vi "ErrorCatcher.vi"(8 "error in":errorcluster, 11 "input String":string) -> (0 "error out":errorcluster)   [LabVIEW 2013]
panel:
  out "concatenated string":string
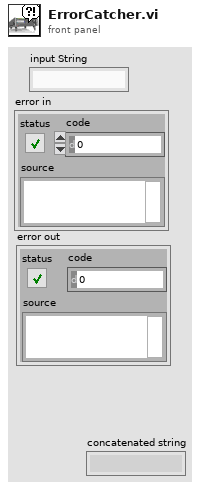
[diagram p1: front panel]
types:
  T1 = cluster{"output string":string, "output string":string}
  T2 = cluster{"output string":string, "output string":string}[]
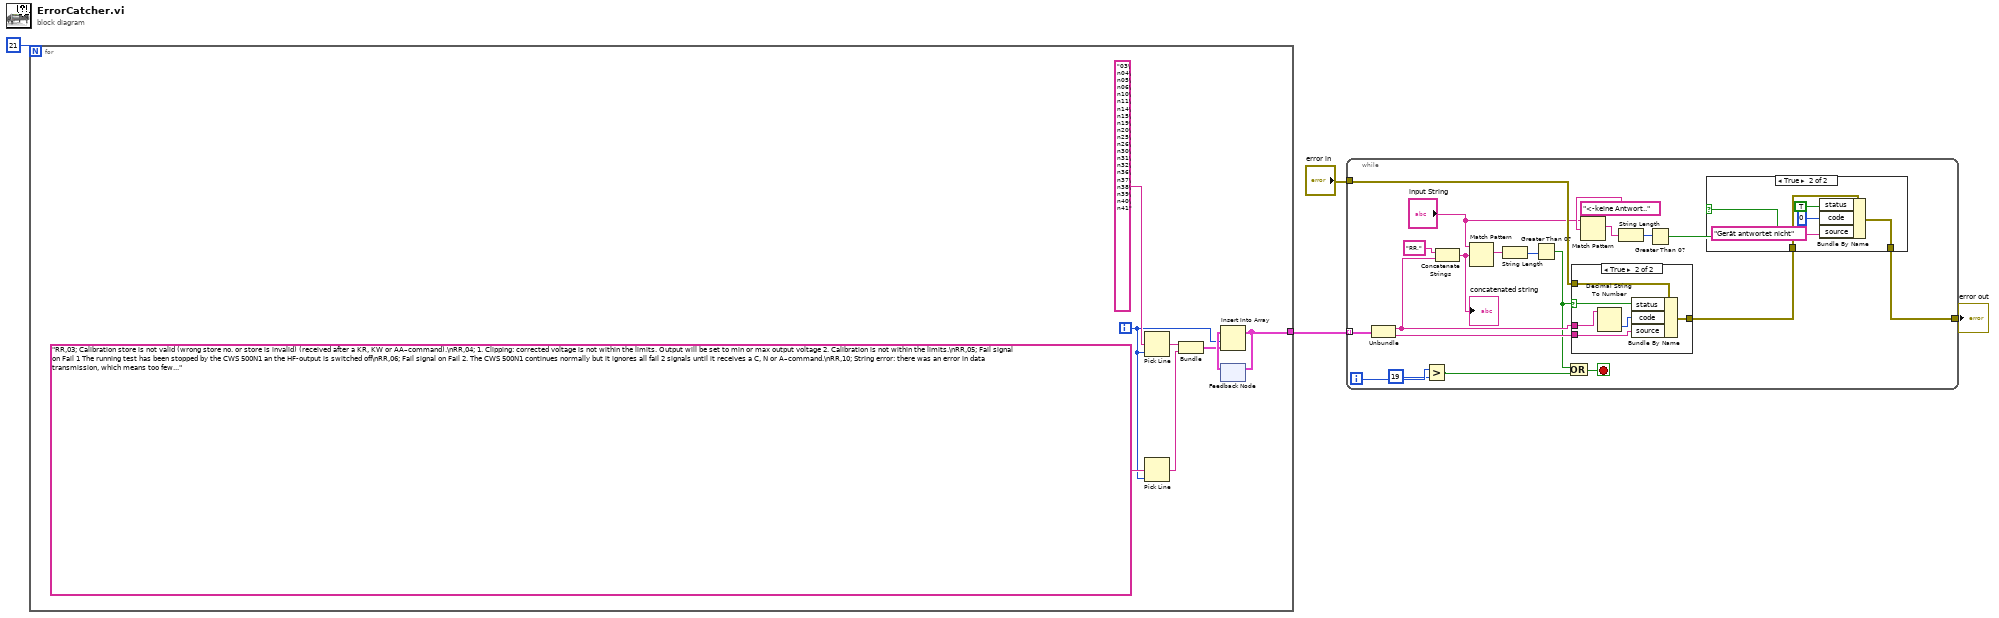
[diagram p0: block diagram]
diagram:
  n1 = for {
    N: 21 -> [_]
    tunnel: [w5] -> w4
    i -> [w7]
    n2 = Pick Line(multi-line string="03\n04\n05\n06\n10\n11\n14\n15\n19\n20\n25\n26\n30\n31\n32\n36\n37\n38\n39\n40\n41", line index=w7) -> (output string=w6:string)  [unwired: 1 in]
    n3 = Pick Line(multi-line string="RR,03; Calibration store is not valid (wrong store no. or store is invalid) (received after a KR, KW or AA–command).\nRR,04; 1. Clipping: corrected voltage is not within the limits. Output will be set to min or max output voltage 2. Calibration is not within the limits.\nRR,05; Fail signal on Fail 1 The running test has been stopped by the CWS 500N1 an the HF-output is switched off\nRR,06; Fail signal on Fail 2. The CWS 500N1 continues normally but it ignores all fail 2 signals until it receives a C, N or A–command.\nRR,10; String error: there was an error in data transmission, which means too few or too many characters or the command is not acceptable.\nRR,11; Test start is not possible or the test has been stopped because TEST ON is not switched on.\nRR,14; One or several values are limited by the CWS 500N1. The parameters are set to their minimum.\nRR,15; Check sum error. The whole command should be sent again.\nRR,19; Internal communication error. Turn off and on the CWS 500N1.\nRR,20; Not correctable limitation error. One or more parameter can not be set to its minimum.\nRR,25; The received calibration data are corrupt (Min-value or Max-value are incorrect or element-no. 265 is not set to 255) (received after a KW–command).\nRR,26; Error on internal Eeprom (write-protected, memory busy) The test routine has been finished correctly using the current monitor. •  This answer will be returned if the test has been invoked by a CN–command with a valid BCI store. parameter Description \nRR,30, V corr , max. current, corr. current; V corr : max. current: corr. current: The factor * 100 between the programmed voltage and the reduced voltage (caused by an overcurrent). The theoretical current at the programmed voltage. The measured current.\nRR,31; Answer to a AA–command if the selected BCI store doesn’t consist of valid data.\nRR,32; BCI store is not valid (the store number is invalid) (received after a KA, KB, KN or KI–command).\nRR,36; BCI store is not valid (there is no valid data in the selected BCI store or the store number is invalid)(received after a KA–command).\nRR,37; The received values for the transfer impedance of the current probe (BCI) are corrupt (Min-value or Max-value are incorrect or element-no. 49 is not set to 65535) (received after a KB–command).\nRR,38; The sent command has no function because there is no PM1000 (current monitor) built in.\nRR,39; Measuring unit not available during a running BCI test\nRR,40; Safety Circuit has been opened. Test stops\nRR,41; PM 40x protection has occured. Test stops", line index=w7) -> (output string=w10:string)  [unwired: 1 in]
    n4 = Bundle("output string"=w6, "output string"=w10) -> (w8:T1)  [unwired: 1 in]
    n5 = feedback #1() -> (w9:T2)  [unwired: 1 in]
    n6 = Insert Into Array(array=w9, index=w7, new element=w8) -> (w5:T2)
    n7 = feedback-in #1(w5) -> ()
  }
  n8 = while {
    tunnel: w4 -> [w32] mode=indexing
    tunnel: "error in" -> [w26]
    tunnel: [w13] -> w1
    i -> [w21]
    stop <- w23 stop-if-true
    n9 = Unbundle(w32) -> ("output string"=w25:string, "output string"=w28:string)
    n10 = Greater?(x=w21, y=19) -> (0:w22:bool)
    n11 = Concatenate Strings("RR,", w25) -> (w27:string)
    "concatenated string" <- w27
    n12 = Match Pattern(string="input String", regular expression=w27) -> (match substring=w31:string)  [unwired: 1 in, 3 out]
    n13 = String Length(string=w31) -> (length=w30:i32)
    n14 = Greater Than 0?(x=w30) -> (x > 0?=w24:bool)
    n15 = Or(x=w24, y=w22) -> (x .or. y?=w23:bool)
    n16 = case shown="True" w24 {
      selector: w24 -> [_ w44]
      tunnel: w25 -> [_ w45]
      tunnel: w28 -> [_ w42]
      tunnel: w26 -> [w39 w41]
      tunnel: [w39 w40] -> w14
      frame False {
      }
      frame True {
        n17 = Decimal String To Number(string=w45) -> (number=w43:i32)  [unwired: 2 in, 1 out]
        n18 = Bundle By Name(cluster=w41, "status"=w44, "code"=w43, "source"=w42) -> (w40:errorcluster)
      }
    }
    n19 = Match Pattern(string="input String", regular expression="<-keine Antwort..") -> (match substring=w18:string)  [unwired: 1 in, 3 out]
    n20 = String Length(string=w18) -> (length=w19:i32)
    n21 = Greater Than 0?(x=w19) -> (x > 0?=w15:bool)
    n22 = case shown="True" w15 {
      tunnel: w14 -> [w33 w37]
      tunnel: [w33 w38] -> w13
      frame False {
      }
      frame True {
        n23 = Bundle By Name(cluster=w37, "status"=TRUE, "code"=0, "source"="Gerät antwortet nicht") -> (w38:errorcluster)
      }
    }
  }
  "error out" <- w1
